vi "Set Theme Mode.vi"(8 "error in":errorcluster, 10 "Theme Mode":u16(ring) items=["Light Theme", "Light Medium Contrast", "Light High Contrast", "Dark Theme", "Dark Medium Contrast", "Dark High Constrast"], 11 "Theme Config in":refnum<class "Theme Config.lvclass">) -> (0 "error out":errorcluster, 3 "Theme Config out":refnum<class "Theme Config.lvclass">)   [LabVIEW 2021, in "Theme Config.lvclass"]
doc: "data member access:\n\nset the theme mode\n\n<b>Code Developed By:</b> +\nDaniel Coons +\nTechnology Service Corporation +\nwww.tsc.com/atcs"
uses:
  Theme Config.lvclass
  Theme Config.lvclass/Theme Config.ctl
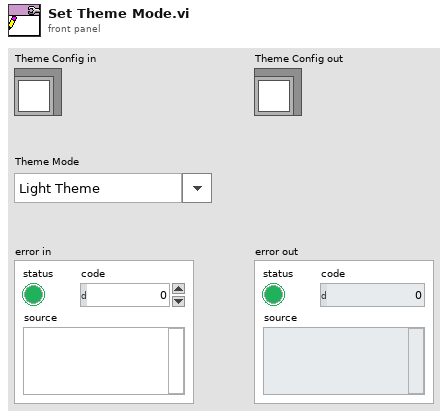
[diagram p1: front panel]
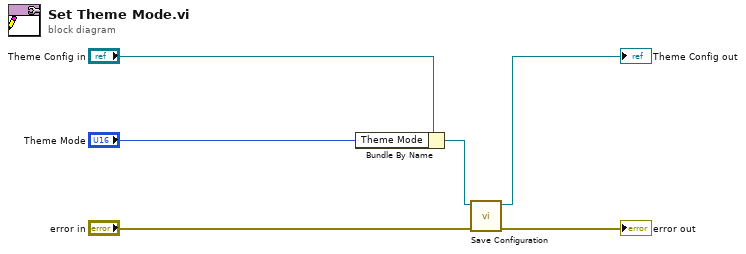
[diagram p0: block diagram]
diagram:
  n1 = Bundle By Name(cluster="Theme Config in", "Theme Mode"="Theme Mode") -> (w2:refnum<class "Theme Config.lvclass">)
  n2 = call "Save Configuration.vi"("error in"="error in", "Theme Config in"=w2) -> ("error out"=→"error out":errorcluster, "Theme Config out"=→"Theme Config out":refnum<class "Theme Config.lvclass">)  [unwired: 8 in]
